vi "example_01_implementation.vi"() -> ()   [LabVIEW 2015, in "lv-post-installer-interface.lvlib"]
uses:
  lv-post-installer-interface.lvlib
  lv-post-installer/public/classes/lv-post-intaller-test/lv-post-installer-test.lvclass
  lv-post-installer/public/classes/lv-post-installer/lv-post-installer.lvclass
panel:
  out "error out":errorcluster
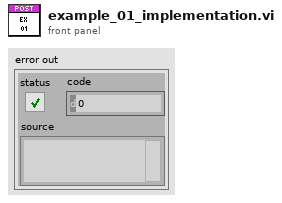
[diagram p1: front panel]
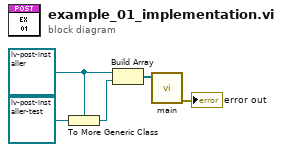
[diagram p0: block diagram]
diagram:
  w3 = refnum<class "lv-post-installer.lvclass"> refnum ("lv-post-installer.lvlib:lv-post-installer.lvclass")
  n1 = To More Generic Class(target class=w3, reference=refnum<class "lv-post-installer-test.lvclass"> refnum ("lv-post-installer.lvlib:lv-post-installer-test.lvclass")) -> (generic class reference=w2:refnum<class "lv-post-installer.lvclass">)
  n2 = Build Array(w3, w2) -> (w5:refnum<class "lv-post-installer.lvclass">[])
  n3 = call "main.vi"("post_installer []"=w5) -> ("error out"=→"error out":errorcluster)  [unwired: 10 in]
